vi "Dba.vi"(11 "VISA Refnum in":refnum<visa-resource-name>) -> (0 "error out":errorcluster, 1 "error out":errorcluster, 2 "connection reference":T1, 3 "VISA Refnum out":refnum<visa-resource-name>)   [LabVIEW 2018]
uses:
  <vilib>/addons/database/Connection.llb/Conn ObjectReference.ctl
  <vilib>/addons/database/Connection.llb/DB Tools Open Connec (Path).vi
  <vilib>/addons/database/NI_Database_API.lvlib
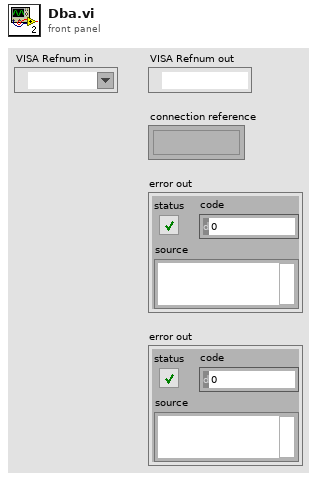
[diagram p1: front panel]
types:
  T1 = typedef "NI_Database_API.lvlib/Conn ObjectReference.ctl" = refnum<k1>
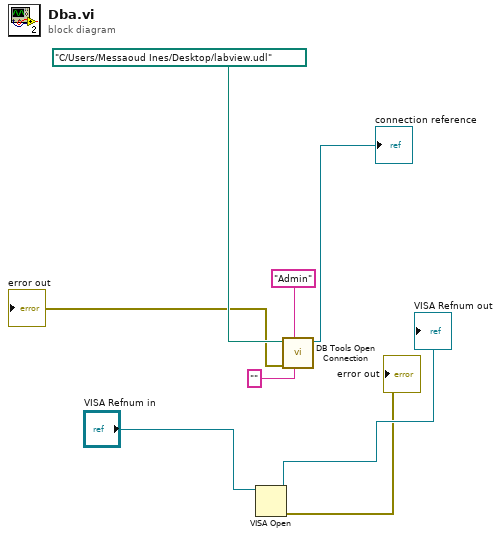
[diagram p0: block diagram]
diagram:
  n1 = VISA Open(VISA resource name="VISA Refnum in") -> (VISA resource name=→"VISA Refnum out":refnum<visa-resource-name>, error out=→"error out":errorcluster)  [unwired: 4 in]
  n2 = call-poly <vilib>:"DB Tools Open Connection.vi"("password"="", "userID"="Admin", "connection information"=path "C:/Users/Messaoud Ines/Desktop/labview.udl") -> ("error out"=→"error out":errorcluster, "connection reference"=→"connection reference":T1)  [unwired: 5 in]
